vi "ACQMODE.vi"(0 "ACQ:NUM":enum16{"4", "16", "64", "128"}(ring), 1 "ACQ MODE":enum16{"SAMPLE", "PEAK DETECT", "AVERAGE"}(ring), 2 "VISA resource name":refnum<visa-resource-name>="GPIB0::7::INSTR") -> ()   [LabVIEW 2011]
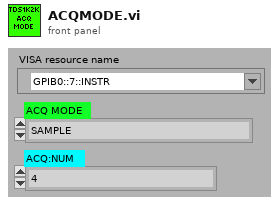
[diagram p1: front panel]
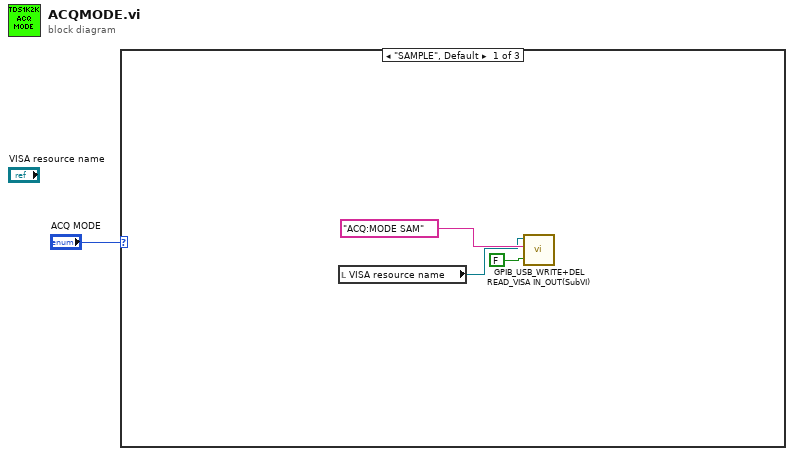
[diagram p0: block diagram]
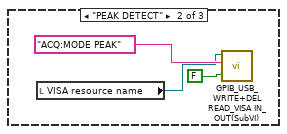
[diagram p2: hidden frame]
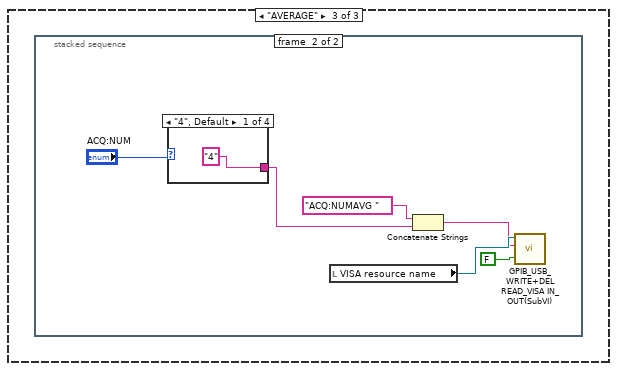
[diagram p3: hidden frame]
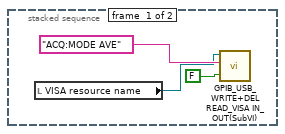
[diagram p4: hidden frame]
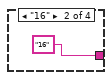
[diagram p5: hidden frame]
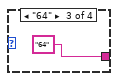
[diagram p6: hidden frame]
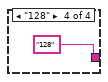
[diagram p7: hidden frame]
diagram:
  n1 = case shown="\"SAMPLE\", Default" "ACQ MODE" {
    frame "SAMPLE", Default {
      n2 = local read "VISA resource name"() -> (w2:refnum<visa-resource-name>)
      n3 = call "GPIB_USB_WRITE+DEL READ_VISA IN_OUT(SubVI).vi"("VISA resource IN"=w2, "GPIB/USB WRITE"="ACQ:MODE SAM" ("GPIB COMMAND"), 4:FALSE ("READ GPIB")) -> ()  [unwired: 3 in, 3 out]
    }
    frame "PEAK DETECT" {
      n4 = local read "VISA resource name"() -> (w5:refnum<visa-resource-name>)
      n5 = call "GPIB_USB_WRITE+DEL READ_VISA IN_OUT(SubVI).vi"("VISA resource IN"=w5, "GPIB/USB WRITE"="ACQ:MODE PEAK" ("GPIB COMMAND"), 4:FALSE ("READ GPIB")) -> ()  [unwired: 3 in, 3 out]
    }
    frame "AVERAGE" {
      n6 = stacked-sequence {
        frame #0 {
          n7 = local read "VISA resource name"() -> (w8:refnum<visa-resource-name>)
          n8 = call "GPIB_USB_WRITE+DEL READ_VISA IN_OUT(SubVI).vi"("VISA resource IN"=w8, "GPIB/USB WRITE"="ACQ:MODE AVE" ("GPIB COMMAND"), 4:FALSE ("READ GPIB")) -> ()  [unwired: 3 in, 3 out]
        }
        frame #1 {
          n9 = case shown="\"4\", Default" "ACQ:NUM" {
            tunnel: ["4" "16" "64" "128"] -> w11
            frame "4", Default {
            }
            frame "16" {
            }
            frame "64" {
            }
            frame "128" {
            }
          }
          n10 = local read "VISA resource name"() -> (w15:refnum<visa-resource-name>)
          n11 = Concatenate Strings("ACQ:NUMAVG " ("GPIB COMMAND"), w11) -> (w14:string)
          n12 = call "GPIB_USB_WRITE+DEL READ_VISA IN_OUT(SubVI).vi"("VISA resource IN"=w15, "GPIB/USB WRITE"=w14, 4:FALSE ("READ GPIB")) -> ()  [unwired: 3 in, 3 out]
        }
      }
    }
  }
